vi "Рассчет времени выполнения.vi"() -> ()   [LabVIEW 2017]
panel:
  out "sqrt(x)":dbl
  out "Скорость выполнения операций":dbl
  out "время работы":dbl
  in  "Количество итераций":i32
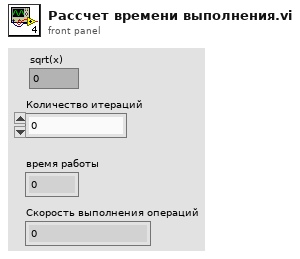
[diagram p1: front panel]
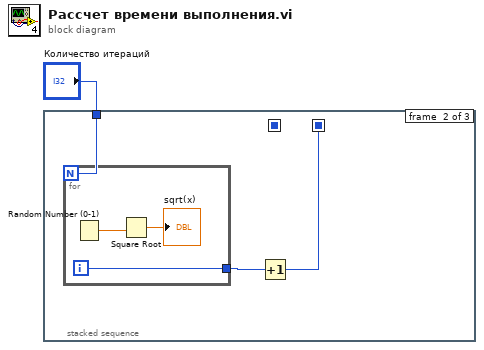
[diagram p0: block diagram]
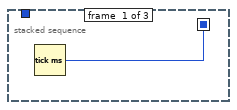
[diagram p2: hidden frame]
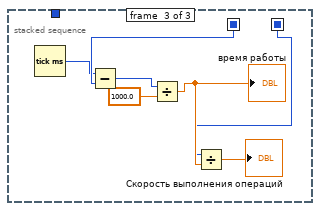
[diagram p3: hidden frame]
diagram:
  n1 = stacked-sequence {
    seq-local: [w2 _ _] -> [_ _ w15]
    seq-local: [_ w3 _] -> [_ _ w10]
    tunnel: "Количество итераций" -> [_ w5 _]
    frame #0 {
      n2 = Tick Count (ms)() -> (millisecond timer value=w2:u32)
    }
    frame #1 {
      n3 = for {
        N: w5 -> [_]
        tunnel: [w7] -> w4
        i -> [w7]
        n4 = Random Number (0-1)() -> (number: 0 to 1=w8:dbl)
        n5 = Square Root(x=w8) -> (sqrt(x)=→"sqrt(x)":dbl)
      }
      n6 = Increment(x=w4) -> (x+1=w3:i32)
    }
    frame #2 {
      n7 = Tick Count (ms)() -> (millisecond timer value=w14:u32)
      n8 = Subtract(x=w14, y=w15) -> (x-y=w12:u32)
      n9 = Divide(x=w12, y=1000.0) -> (x/y=w11:dbl)
      "время работы" <- w11
      n10 = Divide(x=w10, y=w11) -> (x/y=→"Скорость выполнения операций":dbl)
    }
  }
